vi "Connect Channels (Multiple).vi"(8 "error in (no error)":errorcluster, 10 "connection list":string, 11 "SLSC Switch in":refnum<class "SLSC Switch.lvclass">) -> (0 "error out":errorcluster, 3 "SLSC Switch out":refnum<class "SLSC Switch.lvclass">)   [LabVIEW 2016, in "SLSC Switch.lvlib" / "SLSC Switch.lvclass"]
doc: "Creates the connections between channels specified in connection list. Specify connections with two endpoints only or the explicit path between two endpoints. SLSC-SWITCH calculates and uses the shortest path between the channels. Refer to Setting Source and Configuration Channels for information about channel usage types. In the event of an error, connecting stops at the point in the list where the error occurred."
uses:
  SLSC Switch.lvclass
  SLSC Switch.lvclass/SLSC Switch.ctl
  <vilib>/SLSC/Unflatten Names (String).vi
  slscsl/slscsl.lvclass
  <vilib>/SLSC/SLSC.lvlib
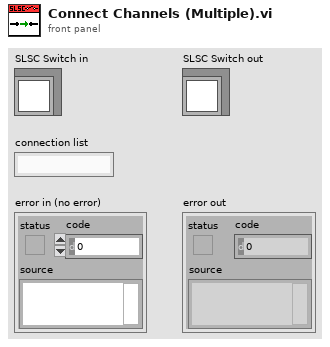
[diagram p1: front panel]
types:
  T1 = typedef "SLSC Switch.lvlib/slscsl.lvclass/SwitchActionsArray.ctl" = T2[]
  T2 = typedef "SLSC Switch.lvlib/slscsl.lvclass/SwitchAction.ctl" = cluster{"index":i32, "RelayAction":T3}
  T3 = typedef "SLSC Switch.lvlib/slscsl.lvclass/RelayAction.ctl" = u32
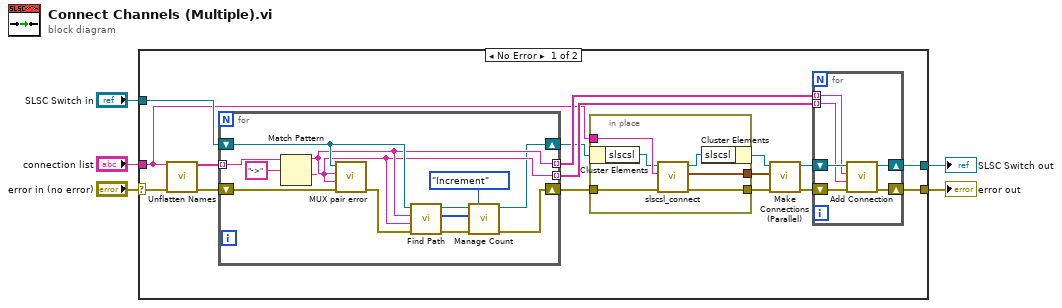
[diagram p0: block diagram]
diagram:
  n1 = case shown="No Error" "error in (no error)" {
    selector: "error in (no error)" -> [w7 w48]
    tunnel: [w13 w48] -> w2
    tunnel: [w14 w47] -> w1
    tunnel: "SLSC Switch in" -> [w18 w47]
    tunnel: "connection list" -> [w9 _]
    frame No Error {
      n2 = call-poly <vilib>:"Unflatten Names.vi"("names in"=w9, "error in (no error)"=w7) -> ("names out"=w8:string[], "error out"=w6:errorcluster)  [unwired: 12 in]
      n3 = for {
        tunnel: w8 -> [w33] mode=indexing
        shift-right: [w22] -> w10
        shift-left: w18 -> [w27]
        shift-right: [w23] -> w15
        shift-left: w6 -> [w32]
        tunnel: [w26] -> w12 mode=indexing
        tunnel: [w25] -> w11 mode=indexing
        n4 = Match Pattern(string=w33, regular expression="->") -> (before substring=w26:string, after substring=w25:string)  [unwired: 1 in, 2 out]
        n5 = call "MUX pair error.vi"("error in (no error)"=w32, "channel 2"=w25, "channel 1"=w26, "SLSC Switch in"=w27) -> ("error out"=w24:errorcluster)  [unwired: 7 in]
        n6 = call "Find Path.vi"("error in (no error)"=w24, "channel 2"=w25, "channel 1"=w26, "SLSC Switch in"=w27) -> ("error out"=w30:errorcluster, "Relay Indexes"=w29:i32[], "SLSC Switch out"=w31:refnum<class "SLSC Switch.lvclass">)  [unwired: 5 in]
        n7 = call "Manage Count.vi"("Inc/Dec"=enum16{"Increment", "Decrement"}."Increment", "error in (no error)"=w30, "Relay Indexes"=w29, "SLSC Switch in"=w31) -> ("error out"=w23:errorcluster, "SLSC Switch out"=w22:refnum<class "SLSC Switch.lvclass">)  [unwired: 5 in, 1 out]
      }
      n8 = in-place {
        in-place-border: w9 -> [w46]
        in-place-border: w15 -> [w45]
        in-place-border: [w44] -> w19
        in-place-border: [w41] -> w20
        n9 = in-place-cluster #1(w10) -> ("slscsl"=w43:refnum<class "slscsl.lvclass">)
        n10 = call "slscsl_connect.vi"("error in (no error)"=w45, "connectionList"=w46, "slscsl in"=w43) -> ("error out"=w44:errorcluster, "switchActionsArray"=w41:T1, "slscsl out"=w42:refnum<class "slscsl.lvclass">)  [unwired: 6 in]
        n11 = in-place-cluster #1("slscsl"=w42) -> (w21:refnum<class "SLSC Switch.lvclass">)
      }
      n12 = call "Make Connections (Parallel).vi"("error in (no error)"=w19, "switchActionsArray"=w20, "SLSC Switch in"=w21) -> ("error out"=w16:errorcluster, "SLSC Switch out"=w17:refnum<class "SLSC Switch.lvclass">)  [unwired: 7 in]
      n13 = for {
        shift-right: [w39] -> w14
        shift-left: w17 -> [w40]
        shift-right: [w37] -> w13
        shift-left: w16 -> [w38]
        tunnel: w12 -> [w36] mode=indexing
        tunnel: w11 -> [w35] mode=indexing
        n14 = call "Add Connection.vi"("error in (no error)"=w38, "channel 2"=w35, "channel 1"=w36, "SLSC Switch in"=w40) -> ("error out"=w37:errorcluster, "SLSC Switch out"=w39:refnum<class "SLSC Switch.lvclass">)  [unwired: 6 in]
      }
    }
    frame Error {
    }
  }
  "error out" <- w2
  "SLSC Switch out" <- w1
